vi "Real Root Finding.vi"() -> ()   [LabVIEW 2023]
doc: "Uses the Polynomial Roots VI to solve for the roots in the following polynomial:\n\na0 + a1 X + a2 X^2 + a3 X^3 + ... = 0\n\nIn this example, a real coefficient array is randomly generated or you can enter it manually. The Polynomial Roots VI solves for the complex roots of the polynomial, and then a utility VI separates the real and complex roots. The polynomial is then plotted over an X range from the smallest real root to the largest real root."
uses:
  <vilib>/Analysis/polynomials.llb/Polynomial Roots (DBL).vi
  <vilib>/Analysis/polynomials.llb/Polynomial Plot (Range).vi
  <vilib>/Analysis/NI_AALPro.lvlib
  <vilib>/Analysis/NI_AALBase.lvlib
panel:
  in  "Roots Found":string="There are %d real roots."
  in  "No roots":string="There are no real roots."
  in  "Orthogonal type":u16(ring) items=["Chebyshev I", "Chebyshev II", "Legendre", "Laguerre", "Hermite", "Associate Laguerre", "Gegenbauer"]
  out "Polynomial":picture
  in  "Coefficient entry":u16(ring)=1 items=["random", "orthogonal"]
  out "P(x) between two real roots":cluster{"Real Roots":dbl[], "P(A)":dbl[]}[](graph)
  out "message":string
  out "Complex Roots":cdb[](array[numeric])
  out "Real Roots":dbl[](array[numeric])
  in  "Order":i32=4
  # "Overview: Demonstrates how to find roots of a polynomial with the Polynomial Roots and Roots Classification VIs.\nRequirements: LabVIEW Full Development System\nInstructions:\n1. Select the Coefficient entry and Order. If you select \"orthogonal\", also select the Orthogonal type of polynomial to generate.\n2. Run the VI.\n3. View the resulting Real Roots, Complex Roots, and P(x) between two real roots."
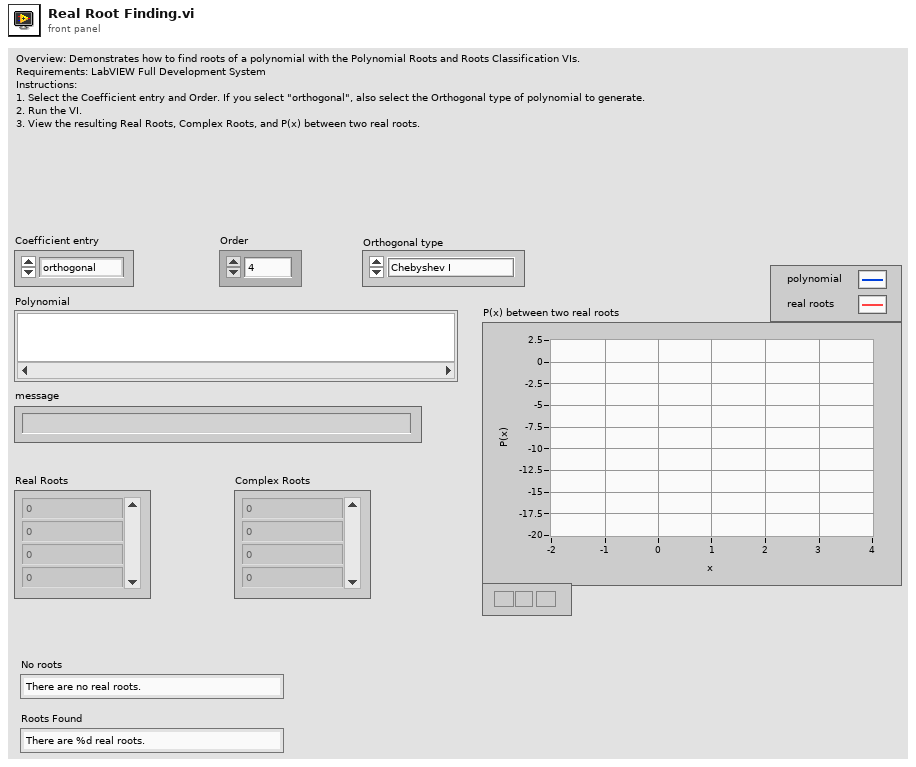
[diagram p1: front panel]
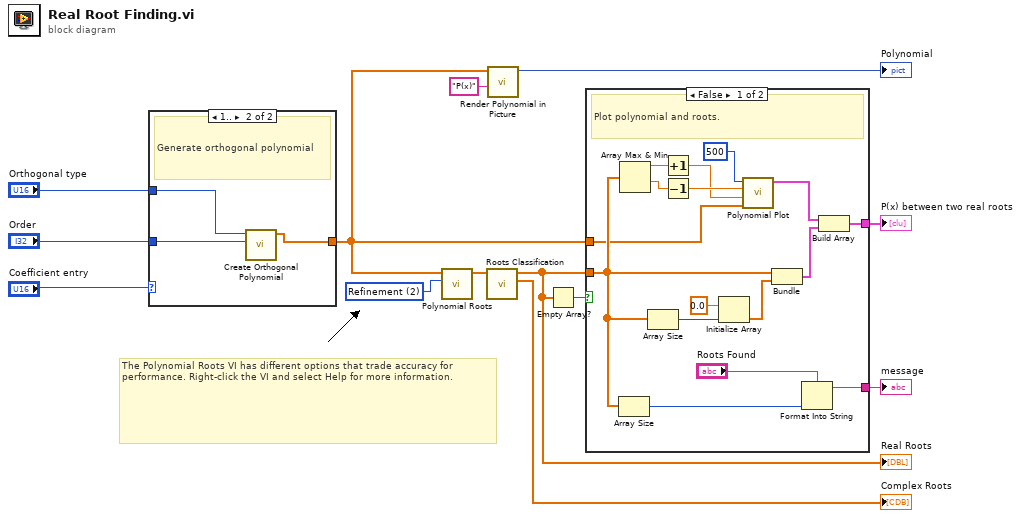
[diagram p0: block diagram]
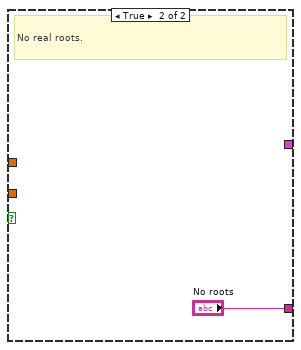
[diagram p2: hidden frame]
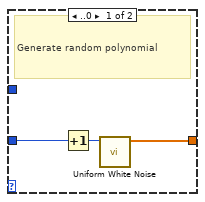
[diagram p3: hidden frame]
diagram:
  w2 = u16 2 items=["General", "Simple Classification", "Refinement", "Advanced Refinement"] ("option")
  # "The Polynomial Roots VI has different options that trade accuracy for performance. Right-click the VI and select Help for more information."
  n1 = case shown="1.." "Coefficient entry" {
    tunnel: [w15 w19] -> w8
    tunnel: "Order" -> [w14 w18]
    tunnel: "Orthogonal type" -> [_ w17]
    frame ..0 {
      # "Generate random polynomial"
      n2 = Increment(x=w14) -> (x+1=w16:i32)
      n3 = call <vilib>:"Uniform White Noise.vi"("samples"=w16) -> ("uniform white noise"=w15:dbl[])  [unwired: 9 in, 1 out]
    }
    frame 1.. {
      # "Generate orthogonal polynomial"
      n4 = call <vilib>:"Create Orthogonal Polynomial.vi"("order"=w18, "type"=w17) -> ("P(x)"=w19:dbl[])  [unwired: 8 in, 1 out]
    }
  }
  n5 = call-poly <vilib>:"Polynomial Roots.vi"("option"=w2, "P(x)"=w8) -> ("Roots"=w13:cdb[])  [unwired: 8 in, 1 out]
  n6 = call <vilib>:"Roots Classification.vi"("Roots"=w13) -> ("Complex Pair Roots"=→"Complex Roots":cdb[], "Real Roots"=w5:dbl[])  [unwired: 7 in, 2 out]
  "Real Roots" <- w5
  n7 = call "Render Polynomial in Picture.vi"("dependent variable"="P(x)", "coefficients"=w8) -> ("rendered equation"=→"Polynomial":picture)  [unwired: 9 in]
  n8 = Empty Array?(array=w5) -> (empty?=w4:bool)
  n9 = case shown="False" w4 {
    tunnel: w5 -> [w29 _]
    tunnel: w8 -> [w25 _]
    tunnel: [w21 "No roots"] -> w10
    tunnel: [w32 _] -> w11
    frame False {
      # "Plot polynomial and roots."
      n10 = Array Size(array=w29) -> (size(s)=w28:i32)
      n11 = Array Max & Min(array=w29) -> (max value=w30:dbl, min value=w31:dbl)  [unwired: 2 out]
      n12 = Array Size(array=w29) -> (size(s)=w33:i32)
      n13 = Increment(x=w30) -> (x+1=w26:dbl)
      n14 = Decrement(x=w31) -> (x-1=w27:dbl)
      n15 = Initialize Array(0.0, w33) -> (w34:dbl[])
      n16 = call-poly <vilib>:"Polynomial Plot.vi"("P(x)"=w25, "end"=w26, "start"=w27, "samples"=500) -> ("polynomial plot"=w24:cluster{"Ramp Pattern":dbl[], "P(A)":dbl[]})  [unwired: 6 in, 1 out]
      n17 = Bundle("Real Roots"=w29, w34) -> (w35:cluster{"Real Roots":dbl[], dbl[]})  [unwired: 1 in]
      n18 = Format Into String(format string="Roots Found", w28) -> (resulting string=w21:string)  [unwired: 2 in, 1 out]
      n19 = Build Array(w24, w35) -> (w32:cluster{"Real Roots":dbl[], "P(A)":dbl[]}[])
    }
    frame True {
      # "No real roots."
    }
  }
  "message" <- w10
  "P(x) between two real roots" <- w11
